vi "LC DB SQL.vi"(7 "Get Record":bool=TRUE, 8 "error in (no error)":errorcluster caption="错误输入（无错误）", 10 "SQL query":string) -> (0 "error out":errorcluster caption="错误输出", 1 "Null?":bool, 2 "Record":string[][](array[string]))   [LabVIEW 2020]
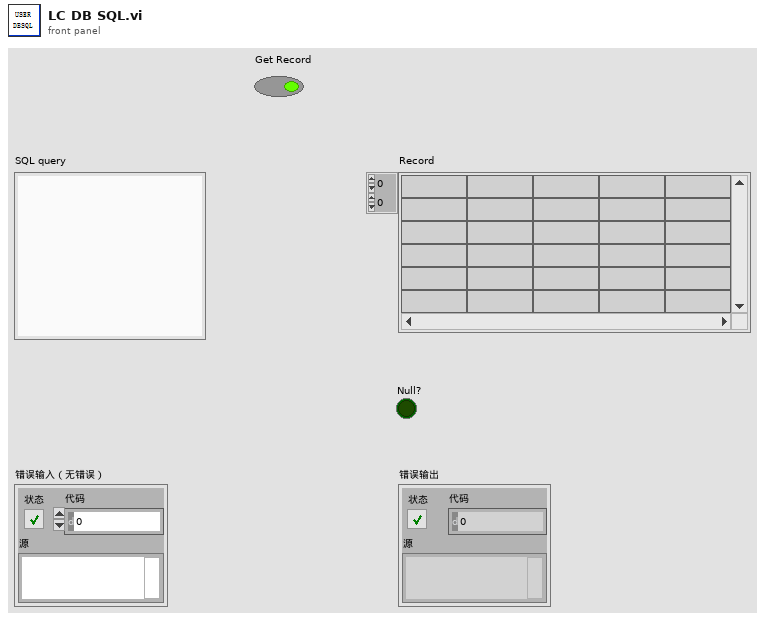
[diagram p1: front panel]
types:
  T1 = typedef "NI_Database_API.lvlib/Conn ObjectReference.ctl" = refnum<k1>
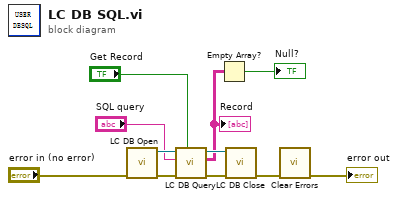
[diagram p0: block diagram]
diagram:
  n1 = call "LC DB Open.vi"("error in (no error)"="error in (no error)") -> ("error out"=w7:errorcluster, "DB Ref Out"=w8:T1)  [unwired: 9 in]
  n2 = call "LC DB Query.vi"("Read?"="Get Record", "error in (no error)"=w7, "SQL query"="SQL query", "DB Ref In"=w8) -> ("error out"=w3:errorcluster, "Data"=w2:string[][], "DB Ref Out"=w4:T1)  [unwired: 5 in]
  "Record" <- w2
  n3 = Empty Array?(array=w2) -> (empty?=→"Null?":bool)
  n4 = call "LC DB Close.vi"("error in (no error)"=w3, "DB Ref In"=w4) -> ("error out"=w11:errorcluster)  [unwired: 9 in]
  n5 = call <vilib>:"Clear Errors.vi"("error in (no error)"=w11) -> ("error out"=→"error out":errorcluster)  [unwired: 5 in, 1 out]
